vi "624WPI_DashboardCreate AVI.vi"(8 "Camera IP":string, 9 "Recording":u16(ring) items=["O", "*", "Open Playback Panel"], 10 "frames per seconds":u32=30, 11 "Image":T1) -> ()   [LabVIEW 2017]
doc: "Depending on Recording Mode, create or add to an AVI file using the Camera IP as part of the name to distinguish different cameras."
uses:
  <vilib>/vision/Image Controls.llb/IMAQ Image.ctl
  <vilib>/Rock Robotics/WPI/Dashboard/WPI_DashboardLogging Global.vi
panel:
  in  "Rec Mode":u16(ring)
  out "Codec Names":string[](array[string])
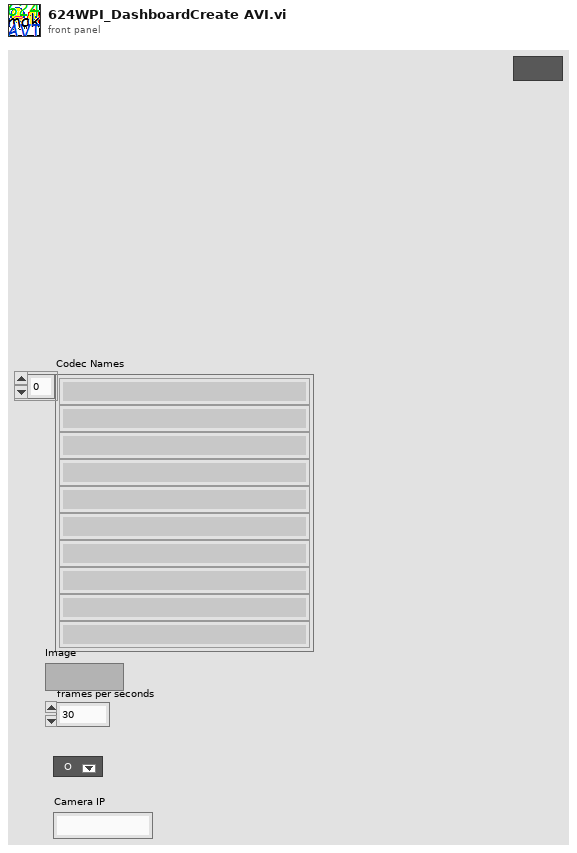
[diagram p1: front panel]
types:
  T1 = typedef "IMAQ Image.ctl" = refnum<image>
  T2 = typedef "IMAQ AVI2 Refnum.ctl" = refnum<k20>
  T3 = cluster{i32, "millisecond timer value":u32, "AVI Refnum (duplicate)":T2}
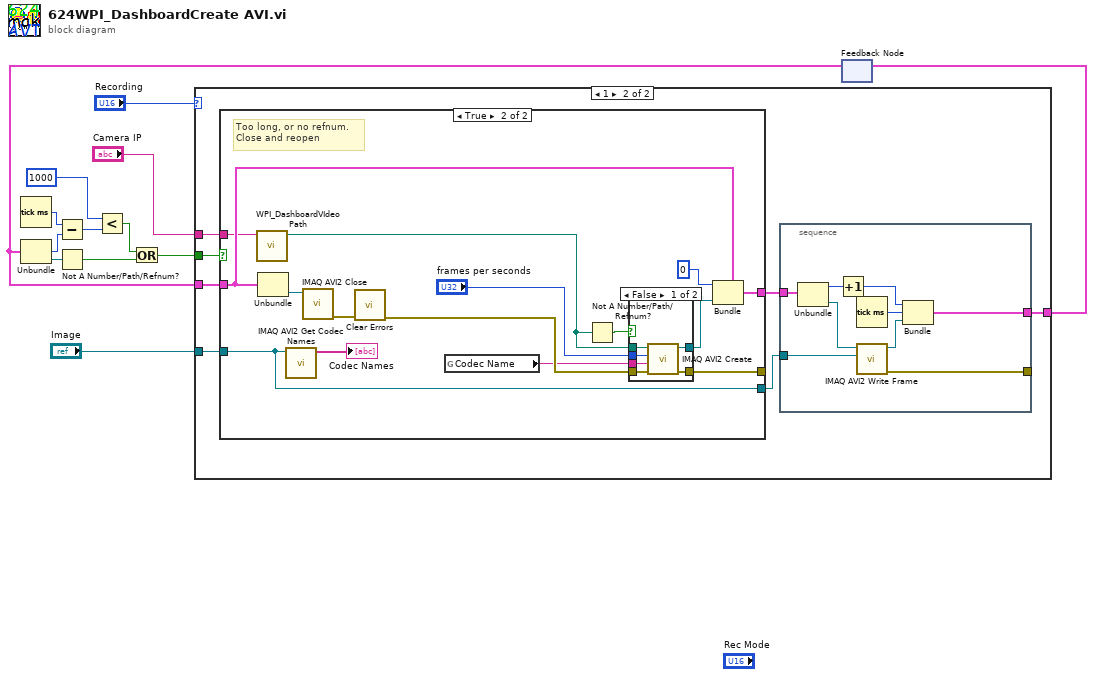
[diagram p0: block diagram]
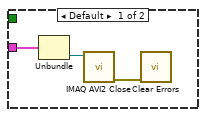
[diagram p2: hidden frame]
diagram:
  n1 = Tick Count (ms)() -> (millisecond timer value=w11:u32)
  n2 = feedback #1() -> (w5:T3)  [unwired: 1 in]
  n3 = Unbundle(w5) -> ("millisecond timer value"=w1:u32, "AVI Refnum (duplicate)"=w2:T2)  [unwired: 1 out]
  n4 = Subtract(x=w11, y=w1) -> (x-y=w9:u32)
  n5 = Not A Number/Path/Refnum?(number/path/refnum=w2) -> (NaN/Path/Refnum?=w10:bool)
  n6 = Less?(x=1000, y=w9) -> (x < y?=w7:bool)
  n7 = Or(x=w7, y=w10) -> (x .or. y?=w6:bool)
  n8 = case shown="1" "Recording" {
    tunnel: "Image" -> [_ w23]
    tunnel: [_ w21] -> w12
    tunnel: w6 -> [_ w20]
    tunnel: w5 -> [w16 w19]
    tunnel: "Camera IP" -> [_ w17]
    frame Default {
      n9 = Unbundle(w16) -> ("AVI Refnum (duplicate)"=w14:T2)  [unwired: 2 out]
      n10 = call "IMAQ AVI2 Close"("AVI Refnum"=w14) -> ("error out"=w15:errorcluster)  [unwired: 10 in]
      n11 = call <vilib>:"Clear Errors.vi"("error in (no error)"=w15) -> ()  [unwired: 5 in, 2 out]
    }
    frame 1 {
      n12 = case shown="True" w20 {
        tunnel: w23 -> [w34 w47]
        tunnel: [w34 w47] -> w22
        tunnel: w19 -> [w33 w44]
        tunnel: [w33 w43] -> w18
        tunnel: w17 -> [_ w42]
        tunnel: [_ w41] -> _
        frame False {
        }
        frame True {
          # "Too long, or no refnum.\nClose and reopen"
          n13 = call <vilib>:"WPI_DashboardVIdeo Path.vi"("Camera IP"=w42) -> ("Video Path"=w39:path)  [unwired: 10 in]
          n14 = Unbundle(w44) -> ("AVI Refnum (duplicate)"=w38:T2)  [unwired: 2 out]
          n15 = call "IMAQ AVI2 Get Codec Names"("Image"=w47) -> ("Codec Names"=→"Codec Names":string[])  [unwired: 9 in, 1 out]
          n16 = call "IMAQ AVI2 Close"("AVI Refnum"=w38) -> ("error out"=w46:errorcluster)  [unwired: 10 in]
          n17 = call <vilib>:"Clear Errors.vi"("error in (no error)"=w46) -> ("error out"=w45:errorcluster)  [unwired: 5 in, 1 out]
          n18 = global read "WPI_DashboardLogging Global.vi" "Codec Name"() -> (w35:string)
          n19 = Not A Number/Path/Refnum?(number/path/refnum=w39) -> (NaN/Path/Refnum?=w40:bool)
          n20 = case shown="False" w40 {
            tunnel: w35 -> [w55 _]
            tunnel: "frames per seconds" -> [w54 _]
            tunnel: w45 -> [w53 w56]
            tunnel: [w52 _] -> w37
            tunnel: [w51 w56] -> w41
            tunnel: w39 -> [w50 _]
            frame False {
              n21 = call "IMAQ AVI2 Create"("error in (no error)"=w53, "Codec"=w55, "Frames Per Second"=w54, "AVI Path"=w50) -> ("error out"=w51:errorcluster, "AVI Refnum"=w52:T2)  [unwired: 6 in]
            }
            frame True {
            }
          }
          n22 = Bundle(cluster=w44, 0, "AVI Refnum (duplicate)"=w37) -> (w43:T3)  [unwired: 1 in]
        }
      }
      n23 = stacked-sequence {
        tunnel: w22 -> [w32]
        tunnel: [w29] -> w21
        tunnel: w18 -> [w28]
        tunnel: [w26] -> _
        frame #0 {
          n24 = Unbundle(w28) -> (w25:i32, "AVI Refnum (duplicate)"=w27:T2)  [unwired: 1 out]
          n25 = Increment(x=w25) -> (x+1=w24:i32)
          n26 = Tick Count (ms)() -> (millisecond timer value=w31:u32)
          n27 = call "IMAQ AVI2 Write Frame"("Image"=w32, "AVI Refnum"=w27) -> ("error out"=w26:errorcluster, "AVI Refnum (duplicate)"=w30:T2)  [unwired: 7 in, 1 out]
          n28 = Bundle(w24, "millisecond timer value"=w31, "AVI Refnum (duplicate)"=w30) -> (w29:T3)  [unwired: 1 in]
        }
      }
    }
  }
  n29 = feedback-in #1(w12) -> ()
